vi "Voorbeeld_Meerdere_Grafieken_XY_graph_Waveform_Graph.vi"() -> ()   [LabVIEW 2019]
panel:
  out "Waveform Chart":cluster{i32, i32}(graph)
  out "Waveform Graph":i32[][](graph)
  out "XY Graph":cluster{i32[], i32[]}[](graph)
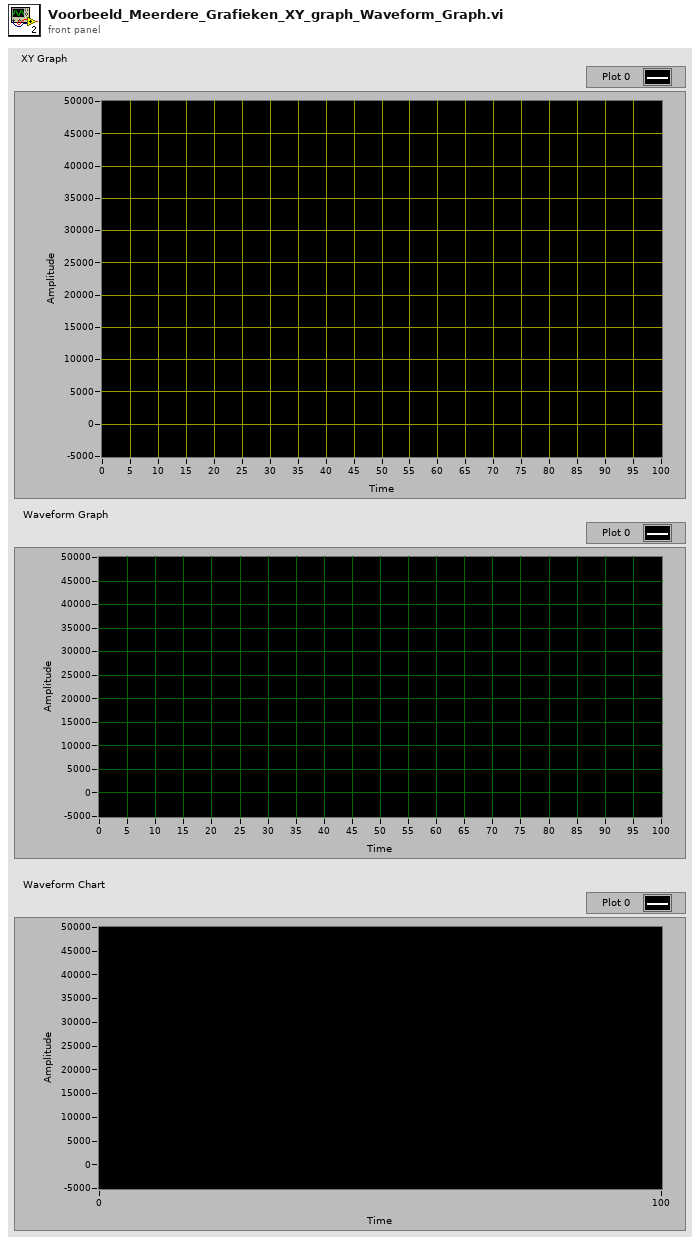
[diagram p1: front panel]
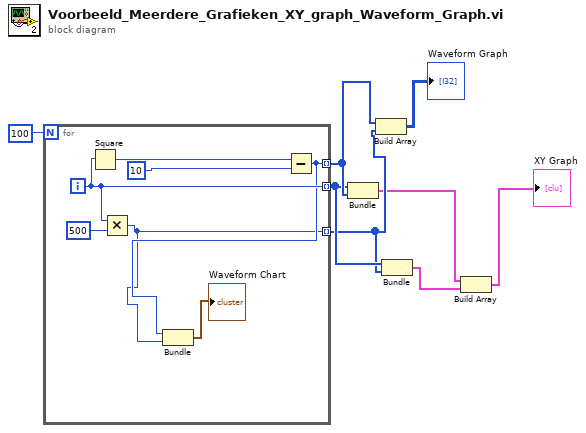
[diagram p0: block diagram]
diagram:
  n1 = for {
    N: 100 -> [_]
    tunnel: [w13] -> w5 mode=indexing
    tunnel: [w11] -> w7 mode=indexing
    tunnel: [w10] -> w4 mode=indexing
    i -> [w13]
    n2 = Square(x=w13) -> (x^2=w15:i32)
    n3 = Multiply(x=w13, y=500) -> (x*y=w10:i32)
    n4 = Subtract(x=w15, y=10) -> (x-y=w11:i32)
    n5 = Bundle(w11, w10) -> (→"Waveform Chart":cluster{i32, i32})  [unwired: 1 in]
  }
  n6 = Bundle(w5, w7) -> (w3:cluster{i32[], i32[]})  [unwired: 1 in]
  n7 = Build Array(w7, w4) -> (→"Waveform Graph":i32[][])
  n8 = Bundle(w5, w4) -> (w2:cluster{i32[], i32[]})  [unwired: 1 in]
  n9 = Build Array(w3, w2) -> (→"XY Graph":cluster{i32[], i32[]}[])
